vi "Resideo Burner Status.vi"(7 "Heat Request":string) -> (3 "Burner":bool)   [LabVIEW 2023]
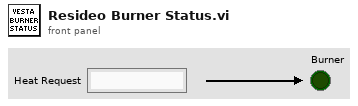
[diagram p1: front panel]
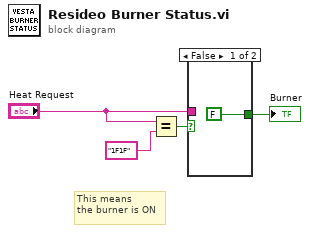
[diagram p0: block diagram]
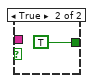
[diagram p2: hidden frame]
diagram:
  # "This means\nthe burner is ON"
  n1 = Equal?(x="Heat Request", y="1F1F") -> (x = y?=w2:bool)
  n2 = case shown="False" w2 {
    tunnel: [FALSE TRUE] -> w4
    tunnel: "Heat Request" -> [_ _]
    frame False {
    }
    frame True {
    }
  }
  "Burner" <- w4
